vi "Software Update HCC Populate Update File List.vi"(8 "Error In":errorcluster, 11 "Stations to Update":bool[](array[boolean])) -> (0 "Error Out":errorcluster, 3 "Update List":i32[](array[numeric]))   [LabVIEW 2016]
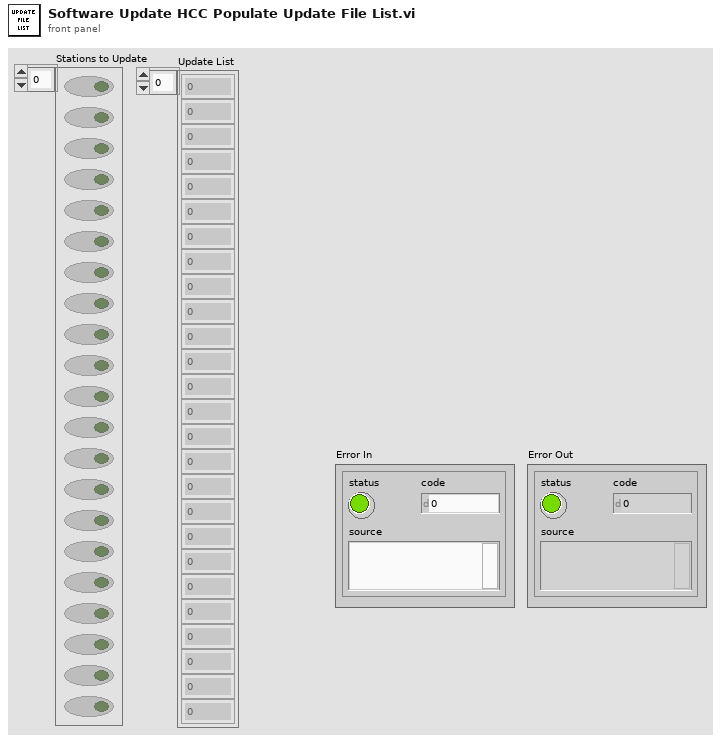
[diagram p1: front panel]
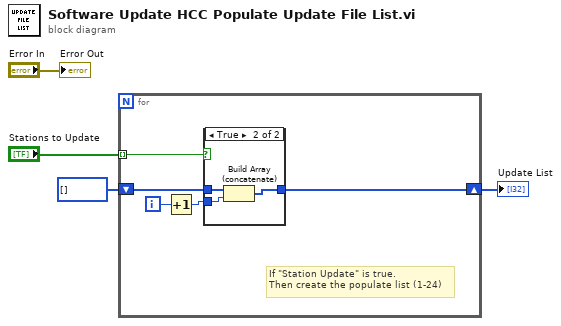
[diagram p0: block diagram]
diagram:
  n1 = for {
    tunnel: "Stations to Update" -> [w5] mode=indexing
    shift-right: [w7] -> w2
    shift-left: i32[] [] -> [w8]
    i -> [w9]
    # "If \"Station Update\" is true.\nThen create the populate list (1-24)"
    n2 = Increment(x=w9) -> (x+1=w6:i32)
    n3 = case shown="True" w5 {
      tunnel: w8 -> [w10 w13]
      tunnel: [w10 w12] -> w7
      tunnel: w6 -> [_ w11]
      frame False {
      }
      frame True {
        n4 = Build Array (concatenate)(w13, w11) -> (w12:i32[])
      }
    }
  }
  "Update List" <- w2
  "Error Out" <- "Error In"
